vi "0-InitialInterfaceControls.vi"(8 "error in (no error)":errorcluster, 11 "AllControls IN":T1) -> (0 "error out":errorcluster, 3 "AllControls Out":T1)   [LabVIEW 2017]
uses:
  Ctrls/AllControls.ctl
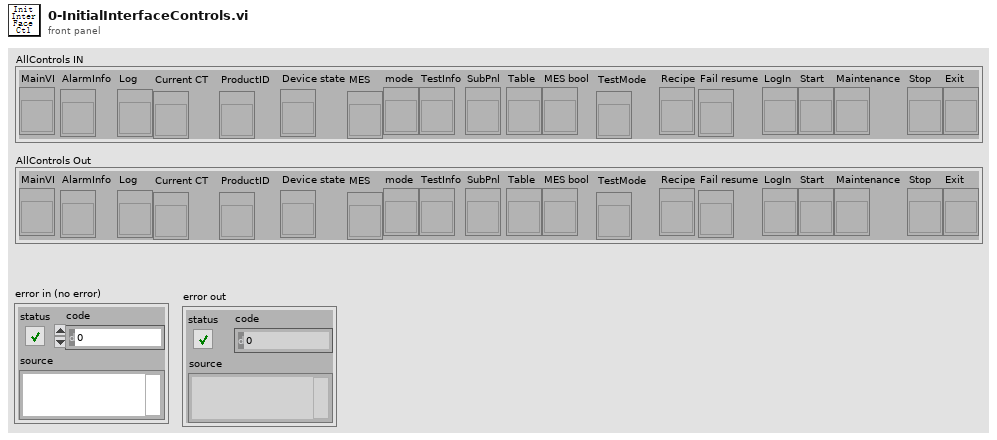
[diagram p1: front panel]
types:
  T1 = typedef "AllControls.ctl" = cluster{"MainVI":refnum<vi>, "AlarmInfo":refnum<vi>, "Log":refnum<vi>, "Current CT":refnum<vi>, "ProductID":refnum<vi>, "Device state":refnum<vi>, "MES":refnum<vi>, "mode":refnum<vi>, "TestInfo":refnum<vi>, "SubPnl":refnum<vi>, "Table":refnum<vi>, "MES bool":refnum<vi>, "TestMode":refnum<vi>, "Recipe":refnum<vi>, "Fail resume":refnum<vi>, "LogIn":refnum<vi>, "Start":refnum<vi>, "Maintenance":refnum<vi>, "Stop":refnum<vi>, "Exit":refnum<vi>}
  T2 = cluster{"Total":i32, "OK":i32, "NG":i32, "Yield":dbl}
  T3 = enum16{"Ini", "Standby", "Running", "Engineering"}
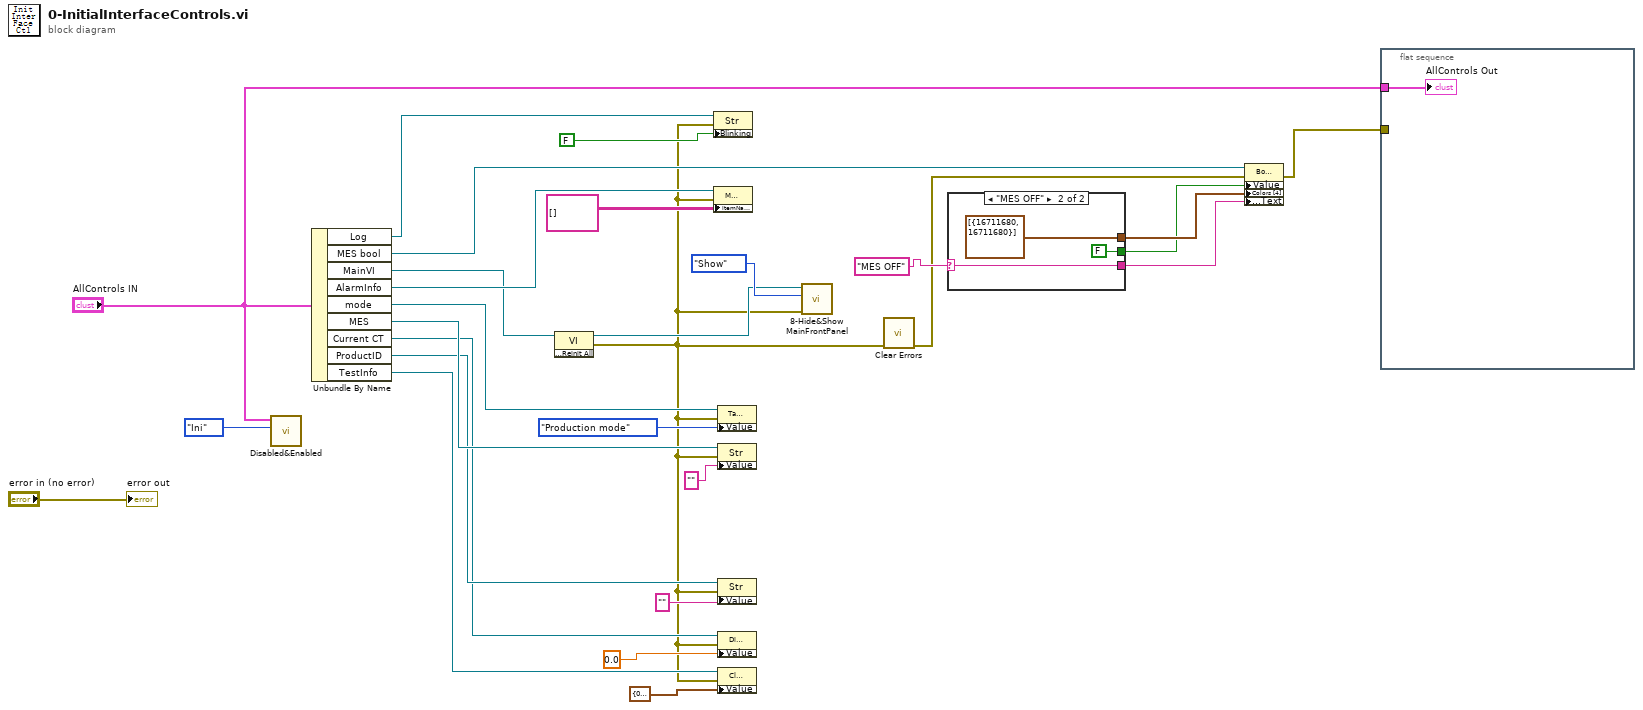
[diagram p0: block diagram]
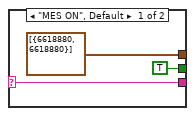
[diagram p2: hidden frame]
diagram:
  n1 = call "Disabled&Enabled.vi"("Mode in"=T3."Ini", "AllControls In"="AllControls IN") -> ()  [unwired: 9 in, 1 out]
  n2 = Unbundle By Name("AllControls IN") -> ("Log"=w11:refnum<vi>, "MES bool"=w6:refnum<vi>, "MainVI"=w2:refnum<vi>, "AlarmInfo"=w25:refnum<vi>, "mode"=w23:refnum<vi>, "MES"=w18:refnum<vi>, "Current CT"=w15:refnum<vi>, "ProductID"=w16:refnum<vi>, "TestInfo"=w13:refnum<vi>)
  n3 = invoke class="VI" method="Default Vals.Reinit All"(reference=w2) -> (reference out=w26:refnum<vi>, error out=w1:errorcluster)  [unwired: 2 in, 1 out]
  n4 = property class="Str"(reference=w11, error in=w1, "Blinking"=FALSE) -> ()  [unwired: 2 out]
  n5 = property class="MCListbox (严格)"(reference=w25, error in=w1, "ItemNames"=string[][] [] ("项名")) -> ()  [unwired: 2 out]
  n6 = property class="TabCtl (严格)"(reference=w23, error in=w1, "Value"=enum32{"Production mode", "Engineering mode"}."Production mode" ("值")) -> ()  [unwired: 2 out]
  n7 = property class="Str"(reference=w18, error in=w1, "Value"="") -> ()  [unwired: 2 out]
  n8 = property class="Str"(reference=w16, error in=w1, "Value"="") -> ()  [unwired: 2 out]
  n9 = property class="DigNum (严格)"(reference=w15, error in=w1, "Value"=0.0) -> ()  [unwired: 2 out]
  n10 = property class="Clust (严格)"(reference=w13, error in=w1, "Value"=T2 {"Total"=0, "OK"=0, "NG"=0, "Yield"=0.0} ("值")) -> ()  [unwired: 2 out]
  n11 = call "8-Hide&Show MainFrontPanel.vi"("error in (no error)"=w1, "Hide&Show"=enum16{"Hide", "Show"}."Show", "This VI"=w26) -> ()  [unwired: 8 in, 1 out]
  n12 = call <vilib>:"Clear Errors.vi"("error in (no error)"=w1) -> ("error out"=w3:errorcluster)  [unwired: 5 in, 1 out]
  n13 = case shown="\"MES OFF\"" "MES OFF" {
    selector: "MES OFF" -> [w29 w32]
    tunnel: [TRUE FALSE] -> w8
    tunnel: [w29 w32] -> w7
    tunnel: [cluster{u32, u32}[] [{6618880, 6618880}] cluster{u32, u32}[] [{16711680, 16711680}]] -> w9
    frame "MES ON", Default {
    }
    frame "MES OFF" {
    }
  }
  n14 = property on="属性节点" class="Bool (严格)"(reference=w6, error in=w3, "Value"=w8, "Colors [4]"=w9, "BoolText.Text"=w7) -> (error out=w4:errorcluster)  [unwired: 1 out]
  n15 = flat-sequence {
    tunnel: "AllControls IN" -> [w35]
    tunnel: w4 -> [_]
    frame #0 {
      "AllControls Out" <- w35
    }
  }
  "error out" <- "error in (no error)"
